vi "BaudDetect-LinColor.vi"(11 "项符号":i32=6) -> (3 "行颜色":u32(colorbox))   [LabVIEW 2011]
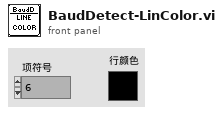
[diagram p1: front panel]
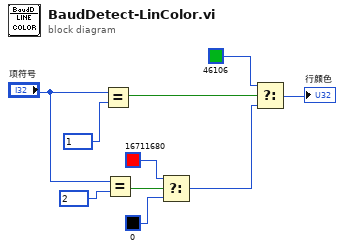
[diagram p0: block diagram]
diagram:
  n1 = Equal?(x="项符号", y=1) -> (x = y?=w9:bool)
  n2 = Equal?(x="项符号", y=2) -> (x = y?=w5:bool)
  n3 = Select(t=u32 16711680, s=w5, f=u32 0) -> (s? t:f=w2:u32)
  n4 = Select(t=u32 46106, s=w9, f=w2) -> (s? t:f=→"行颜色":u32)
